vi "Fetch Tab Pages.vi"(5 "Max Level (10)":i32, 6 "Current Level (0)":i32, 7 "Draw Controls":T4, 8 "error in (no error)":errorcluster, 9 "Pages":refnum<vi>[](array[refnum]), 10 "Parent":string, 11 "Tab Ref in":refnum<vi>) -> (0 "error out":errorcluster, 2 "Results":T1[](array[typedef]), 3 "Tab Ref out":refnum<vi>)   [LabVIEW 2023, in "VIDoc Parsing.lvlib"]
uses:
  VIDoc Parsing.lvlib
  Settings/Parser Settings/Draw Controls Cluster.ctl
  Settings/Parser Settings/Draw Option Enum.ctl
  TypeDefs/Controls Info Cluster.ctl
  <vilib>/picture/picture.llb/imagedata.ctl
  <vilib>/Utility/miscctls.llb/LVKeyTypeDef.ctl
  65cc6c1e-4fa3-40c4-af1b-ec562817ce9d.vi
  Settings/Parser Settings/Parser Settings.lvclass
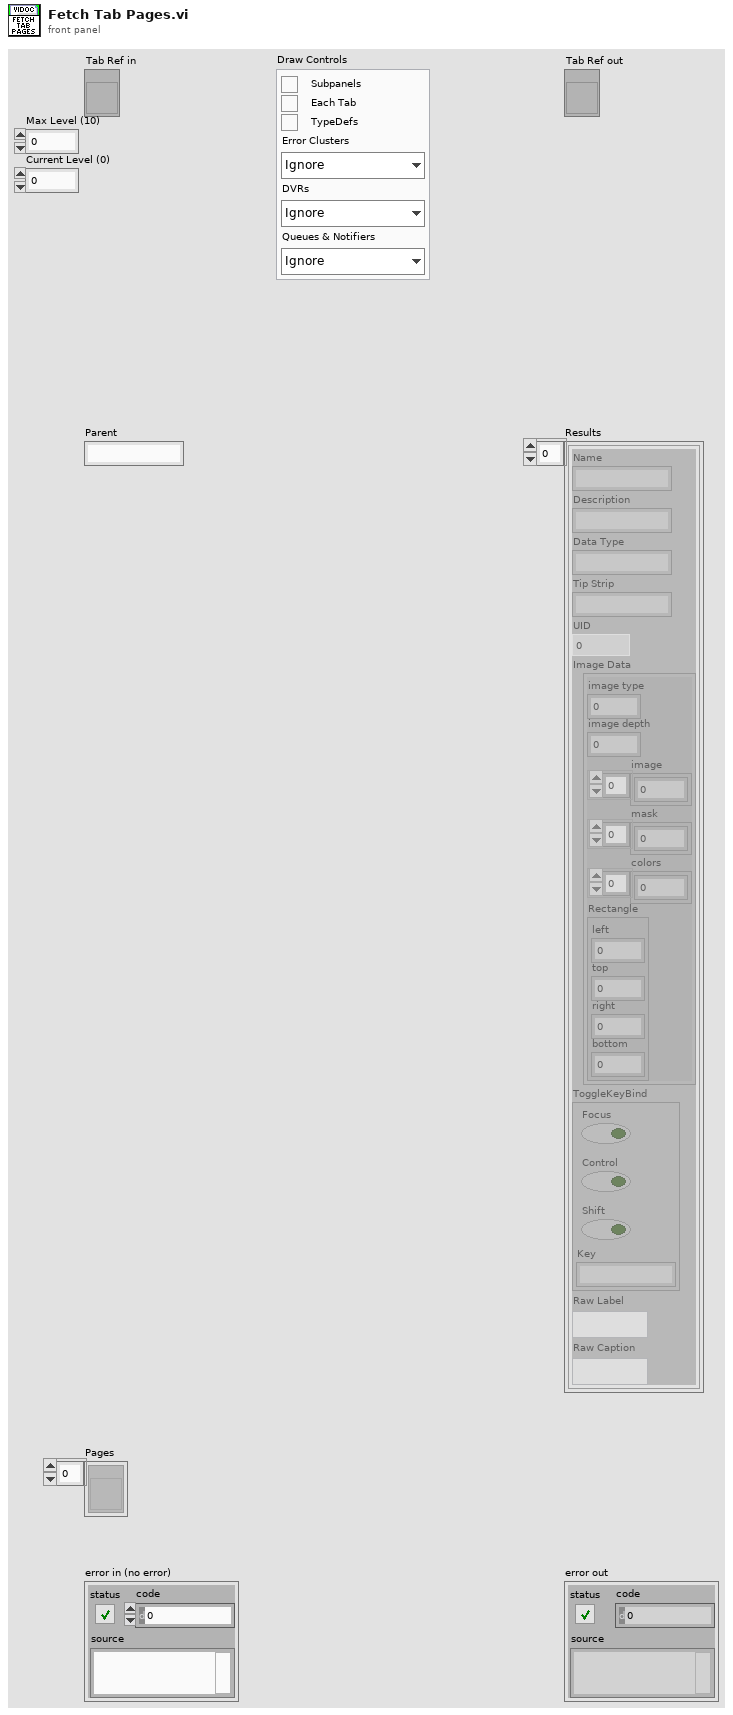
[diagram p1: front panel]
types:
  T1 = typedef "VIDoc Parsing.lvlib/Controls Info Cluster.ctl" = cluster{"Name":string, "Description":string, "Data Type":string, "Tip Strip":string, "UID":i32, "Image Data":T2, "ToggleKeyBind":T3, "Raw Label":string, "Raw Caption":string}
  T2 = typedef "imagedata.ctl" = cluster{"image type":i32, "image depth":i32, "image":u8[], "mask":u8[], "colors":u32[], "Rectangle":cluster{"left":i16, "top":i16, "right":i16, "bottom":i16}}
  T3 = typedef "LVKeyTypeDef.ctl" = cluster{"Focus":bool, "Control":bool, "Shift":bool, "Key":string}
  T4 = typedef "VIDoc Parsing.lvlib/Parser Settings.lvclass/Draw Controls Cluster.ctl" = cluster{"Subpanels":bool, "Tabs":bool, "TypeDefs":bool, "Error Clusters":T5, "DVRs":T5, "Queues & Notifiers":T5}
  T5 = typedef "VIDoc Parsing.lvlib/Parser Settings.lvclass/Draw Option Enum.ctl" = enum16{"Ignore", "Draw", "Draw + Contents"}
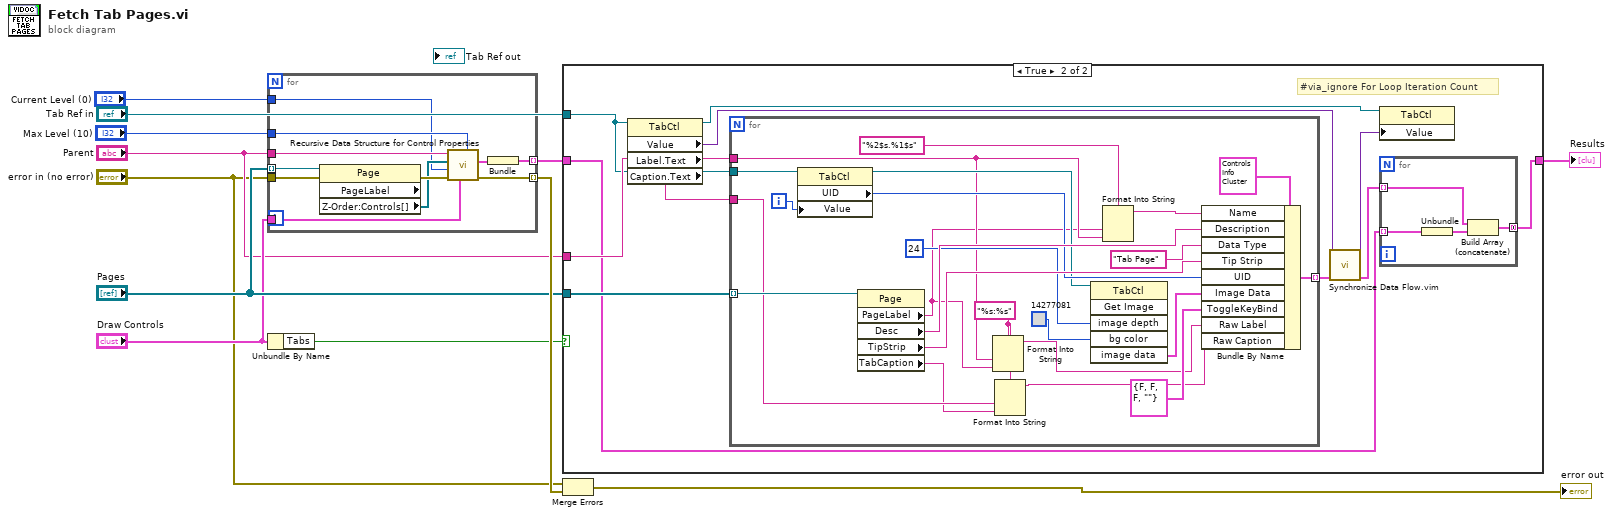
[diagram p0: block diagram]
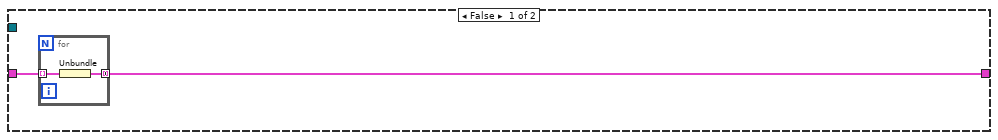
[diagram p2: hidden frame]
diagram:
  n1 = for {
    tunnel: "error in (no error)" -> [w23]
    tunnel: [w20] -> w12 mode=indexing
    tunnel: "Parent" -> [w16]
    tunnel: "Draw Controls" -> [w18]
    tunnel: "Pages" -> [w22] mode=indexing
    tunnel: [w21] -> w5 mode=indexing
    tunnel: "Max Level (10)" -> [w14]
    tunnel: "Current Level (0)" -> [w13]
    n2 = property class="Page" props=["PageLabel", "Z-Order:Controls[]"](reference=w22, error in=w23) -> (error out=w19:errorcluster, "Z-Order:Controls[]"=w17:refnum<vi>[])  [unwired: 2 out]
    n3 = call "Recursive Data Structure for Control Properties.vi"("Max Level (10)"=w14, "Draw Controls"=w18, "error in"=w19, "Current Level (0)"=w13, "Controls[]"=w17, "Parent's name"=w16) -> ("error out"=w20:errorcluster, "Results"=w15:T1[])  [unwired: 4 in]
    n4 = Bundle("Results"=w15) -> (w21:cluster{"Results":T1[]})  [unwired: 1 in]
  }
  n5 = Unbundle By Name("Draw Controls") -> ("Tabs"=w8:bool)
  n6 = case shown="True" w8 {
    tunnel: "Pages" -> [_ w38]
    tunnel: "Parent" -> [_ w37]
    tunnel: "Tab Ref in" -> [_ w36]
    tunnel: w5 -> [w25 w30]
    tunnel: [w24 w29] -> w4
    frame False {
      n7 = for {
        tunnel: w25 -> [w27] mode=indexing
        tunnel: [w26] -> w24 mode=concatenating
        n8 = Unbundle(w27) -> ("Results"=w26:T1[])
      }
    }
    frame True {
      # "#via_ignore For Loop Iteration Count"
      n9 = property class="TabCtl" props=["Value", "Label", "Text", "Caption", "Text"](reference=w36) -> (reference out=w32:refnum<vi>, "Value"=w35:variant, "Caption.Text"=w28:string)  [unwired: 1 in, 2 out]
      n10 = for {
        tunnel: w38 -> [w54] mode=indexing
        tunnel: [w64] -> w33 mode=indexing
        tunnel: w37 -> [w50]
        tunnel: w36 -> [w58]
        tunnel: w28 -> [w48]
        i -> [w56]
        w44 = "%s:%s" ("format string")
        n11 = property class="TabCtl"(reference=w58, "Value"=w56) -> (reference out=w53:refnum<vi>, "UID"=w57:i32)  [unwired: 1 in, 1 out]
        n12 = property class="Page"(reference=w54) -> ("PageLabel"=w49:string, "Desc"=w61:string, "TipStrip"=w59:string, "TabCaption"=w47:string)  [unwired: 1 in, 2 out]
        n13 = Format Into String(format string=w44, w50, w49) -> (resulting string=w46:string)  [unwired: 2 in, 1 out]
        n14 = Format Into String(format string=w44, w48, w47) -> (resulting string=w45:string)  [unwired: 2 in, 1 out]
        n15 = invoke class="TabCtl" method="Get Image"(reference=w53, "image depth"=24 ("Image Depth"), "bg color"=u32 14277081 ("Color Box")) -> ("image data"=w52:T2)  [unwired: 3 in, 5 out]
        n16 = Format Into String(format string="%2$s.%1$s", w49, w50) -> (resulting string=w62:string)  [unwired: 2 in, 1 out]
        n17 = Bundle By Name(cluster=T1 {"Name"="", "Description"="", "Data Type"="", "Tip Strip"="", "UID"=0, "Image Data"={"image type"=0, "image depth"=0, "image"=[], "mask"=[], "colors"=[], "Rectangle"={"left"=0, "top"=0, "right"=0, "bottom"=0}}, "ToggleKeyBind"={"Focus"=FALSE, "Control"=FALSE, "Shift"=FALSE, "Key"=""}, "Raw Label"="", "Raw Caption"=""}, "Name"=w62, "Description"=w61, "Data Type"="Tab Page", "Tip Strip"=w59, "UID"=w57, "Image Data"=w52, "ToggleKeyBind"=T3 {"Focus"=FALSE, "Control"=FALSE, "Shift"=FALSE, "Key"=""}, "Raw Label"=w46, "Raw Caption"=w45) -> (w64:T1)
      }
      n18 = call "Synchronize Data Flow.vim"("input 4"=w33, "input 1"=w35) -> ("output 4"=w31:T1[], "output 1"=w34:variant)  [unwired: 2 in, 2 out]
      n19 = property class="TabCtl"(reference=w32, "Value"=w34) -> ()  [unwired: 1 in, 2 out]
      n20 = for {
        tunnel: w31 -> [w41] mode=indexing
        tunnel: w30 -> [w42] mode=indexing
        tunnel: [w39] -> w29 mode=concatenating
        n21 = Unbundle(w42) -> ("Results"=w40:T1[])
        n22 = Build Array (concatenate)(w41, w40) -> (w39:T1[])
      }
    }
  }
  "Results" <- w4
  n23 = Merge Errors("error in (no error)", w12) -> (→"error out":errorcluster)
